vi "C37 Disconnect from PDC.vi"(8 "error in (no error)":errorcluster, 11 "Pseudo PDC ID":i32) -> (0 "error out":errorcluster)   [LabVIEW 2013, in "C37118-DLL.lvlib"]
uses:
  C37118-DLL.lvlib
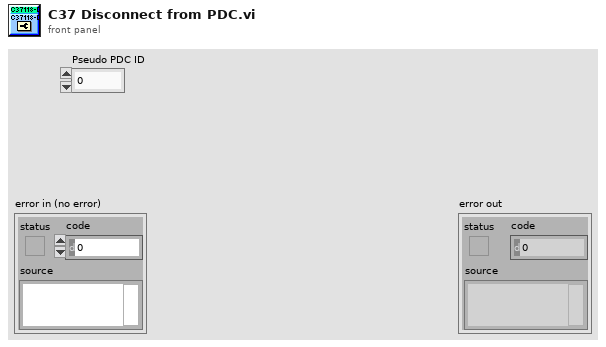
[diagram p1: front panel]
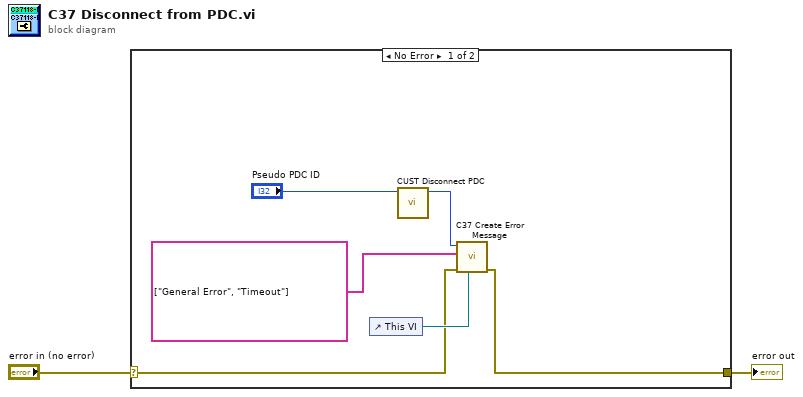
[diagram p0: block diagram]
diagram:
  n1 = case shown="No Error" "error in (no error)" {
    selector: "error in (no error)" -> [w7 w9]
    tunnel: [w6 w9] -> w2
    frame No Error {
      n2 = control-ref of="This VI"() -> (w8:refnum<vi>)
      n3 = call "CUST Disconnect PDC.vi"("pseudoPdcId"="Pseudo PDC ID") -> ("function return"=w4:i32)  [unwired: 10 in]
      n4 = call "C37 Create Error Message.vi"("VI Reference"=w8, "error in (no error)"=w7, "Error Messages"=string[] ["General Error", "Timeout"], "function return"=w4) -> ("error out"=w6:errorcluster)  [unwired: 7 in]
    }
    frame Error {
    }
  }
  "error out" <- w2
